vi "Compiled Help Menu Wizard.vi"   [LabVIEW 2015]
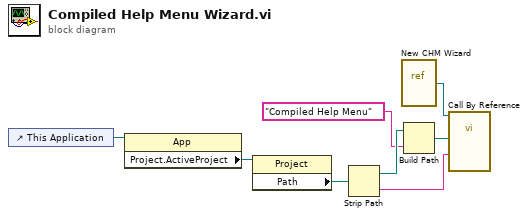
[diagram p0: block diagram]
diagram:
  n1 = control-ref of="This Application"() -> (w7:refnum<vi>)
  n2 = property class="App"(reference=w7) -> ("Project.ActiveProject"=w6:refnum<vi>)  [unwired: 1 in, 2 out]
  n3 = property class="Project"(reference=w6) -> ("Path"=w5:path)  [unwired: 1 in, 2 out]
  n4 = Strip Path(path=w5) -> (stripped path=w4:path, name=w1:string)
  n5 = vi-ref "New CHM Wizard.vi"() -> (w8:refnum<vi>)
  n6 = Build Path(base path=w4, name or relative path="Compiled Help Menu") -> (appended path=w2:path)
  n7 = call-by-ref "?"(reference=w8, "Title"=w1, "Base CHM Directory"=w2) -> ()  [unwired: 11 in, 2 out]
